vi "backup documentation 1.vi"   [LabVIEW 2017]
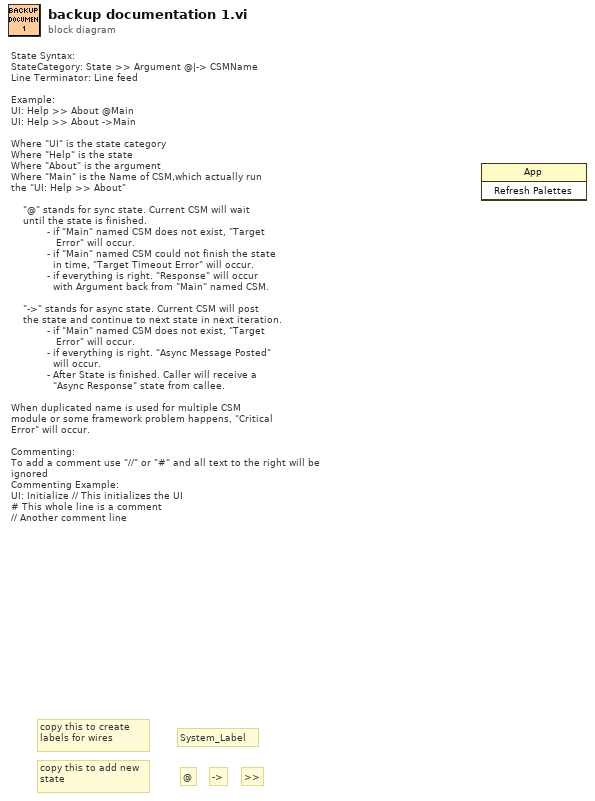
[diagram p0: block diagram]
diagram:
  # "copy this to add new state"
  # ">>"
  # "->"
  # "@"
  # "State Syntax:\nStateCategory: State >> Argument @|-> CSMName\nLine Terminator: Line feed\n\nExample:\nUI: Help >> About @Main\nUI: Help >> About ->Main\n\nWhere \"UI\" is the state category\nWhere \"Help\" is the state\nWhere \"About\" is the argument\nWhere \"Main\" is the Name of CSM,which actually run \nthe \"UI: Help >> About\"\n\n    \"@\" stands for sync state. Current CSM will wait \n    until the state is finished. \n            - if \"Main\" named CSM does not exist, \"Target \n               Error\" will occur.\n            - if \"Main\" named CSM could not finish the state \n              in time, \"Target Timeout Error\" will occur.\n            - if everything is right. \"Response\" will occur \n              with Argument back from \"Main\" named CSM. \n\n    \"->\" stands for async state. Current CSM will post \n    the state and continue to next state in next iteration.\n            - if \"Main\" named CSM does not exist, \"Target \n               Error\" will occur.\n            - if everything is right. \"Async Message Posted\"\n              will occur.\n            - After State is finished. Caller will receive a \n              \"Async Response\" state from callee.\n\nWhen duplicated name is used for multiple CSM \nmodule or some framework problem happens, \"Critical \nError\" will occur.\n\nCommenting:\nTo add a comment use \"//\" or \"#\" and all text to the right will be ignored\nCommenting Example:\nUI: Initialize // This initializes the UI\n# This whole line is a comment\n// Another comment line"
  # "copy this to create labels for wires"
  # "System_Label"
  n1 = invoke class="App" method="Refresh Palettes"() -> ()  [unwired: 3 in, 3 out]
